vi "Round.vi"(1 "Digits":i32=2, 2 "A":T1={"Array Num"=[1, 2, 3], "Decimal Index"=0, "stop"=FALSE}) -> (0 "A rounded to Digits":T1={"Array Num"=[1, 2, 3], "Decimal Index"=0, "stop"=FALSE})   [LabVIEW 2025]
uses:
  Number.ctl
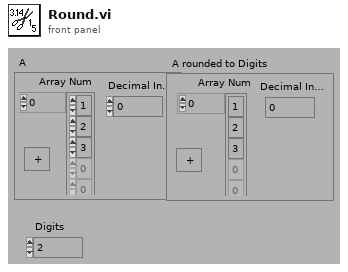
[diagram p1: front panel]
types:
  T1 = typedef "Number.ctl" = cluster{"Array Num":i8[], "Decimal Index":i32, "stop":bool}
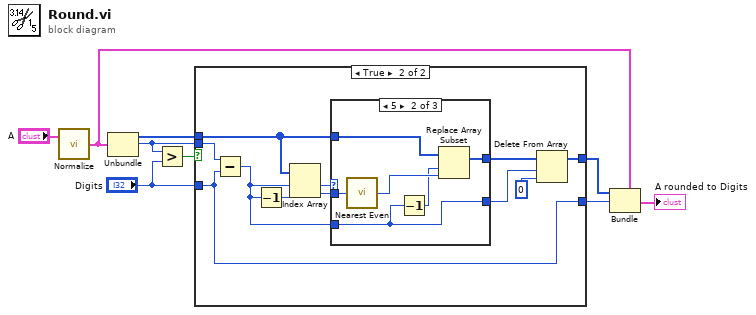
[diagram p0: block diagram]
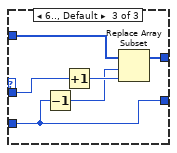
[diagram p4: hidden frame]
diagram:
  n1 = call "Normalize.vi"("A"="A") -> ("Normalized A"=w7:T1)  [unwired: 1 in]
  n2 = Unbundle(w7) -> ("Array Num"=w5:i8[], "Decimal Index"=w1:i32)  [unwired: 1 out]
  n3 = Greater?(x=w1, y="Digits") -> (0:w6:bool)
  n4 = case shown="True" w6 {
    tunnel: w5 -> [w11 w21]
    tunnel: [w11 w22] -> w8
    tunnel: "Digits" -> [_ w12]
    tunnel: [w10 w12] -> w2
    tunnel: w1 -> [w10 w17]
    frame False {
    }
    frame True {
      n5 = Subtract(x=w17, y=w12) -> (x-y=w16:i32)
      n6 = Decrement(x=w16) -> (x-1=w18:i32)
      n7 = Index Array(array=w21, index #1=w16, index #2=w18) -> (element #1=w20:i8, element #2=w19:i8)
      n8 = case shown="5" w20 {
        tunnel: w21 -> [w24 w27 w36]
        tunnel: [w24 w30 w34] -> w15
        tunnel: w16 -> [w23 w26 w32]
        tunnel: [w23 w26 w32] -> w14
        tunnel: w19 -> [_ w28 w31]
        frame ..4 {
        }
        frame 5 {
          n9 = call "Nearest Even.vi"("digit"=w28) -> ("Rounded to even"=w29:i8)
          n10 = Decrement(x=w26) -> (x-1=w25:i32)
          n11 = Replace Array Subset(array=w27, new element=w29, index=w25) -> (w30:i8[])
        }
        frame 6.., Default {
          n12 = Decrement(x=w32) -> (x-1=w33:i32)
          n13 = Increment(x=w31) -> (x+1=w35:i8)
          n14 = Replace Array Subset(array=w36, new element=w35, index=w33) -> (w34:i8[])
        }
      }
      n15 = Delete From Array(array=w15, length=w14, index=0) -> (array with subset deleted=w22:i8[])  [unwired: 1 out]
    }
  }
  n16 = Bundle(cluster=w7, "Array Num"=w8, "Decimal Index"=w2) -> (→"A rounded to Digits":T1)  [unwired: 1 in]
